vi "Set Output DT.vi"(0 "Scaling configuration in":refnum<class "Scaling configuration.lvclass">, 5 "Scale Data Type":T1, 7 "Scale Index":i32, 9 "Mapping Index":i32, 11 "error in (no error)":errorcluster) -> (4 "Scaling configuration out":refnum<class "Scaling configuration.lvclass">, 15 "error out":errorcluster)   [LabVIEW 2013, in "Scaling configuration.lvclass"]
uses:
  Scaling configuration.lvclass
  controls/scale data types.ctl
  Scaling configuration.lvclass/Scaling configuration.ctl
  <vilib>/NI/Tag Bus/tag/tag descriptor.lvclass/tag descriptor.ctl
  <vilib>/NI/Tag Bus/tag/tag descriptor.lvclass
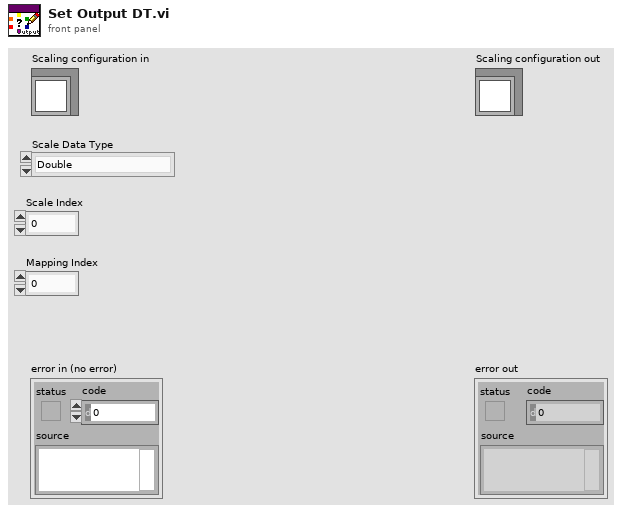
[diagram p1: front panel]
types:
  T1 = typedef "Scaling configuration.lvclass/scale data types.ctl" = enum16{"Double", "Single", "I64", "I32", "I16", "I8", "U64", "U32", "U16", "U8", "Boolean (0,1)"}
  T2 = cluster{"mappings":cluster{"input channel":refnum<class "TBM channel.lvclass">, "output channel":refnum<class "TBM channel.lvclass">, "input data type":T1, "output data type":T1}[], "name":string}[]
  T3 = cluster{"mappings":cluster{"input channel":refnum<class "TBM channel.lvclass">, "output channel":refnum<class "TBM channel.lvclass">, "input data type":T1, "output data type":T1}[], "name":string}
  T4 = cluster{"input channel":refnum<class "TBM channel.lvclass">, "output channel":refnum<class "TBM channel.lvclass">, "input data type":T1, "output data type":T1}[]
  T5 = cluster{"input channel":refnum<class "TBM channel.lvclass">, "output channel":refnum<class "TBM channel.lvclass">, "input data type":T1, "output data type":T1}
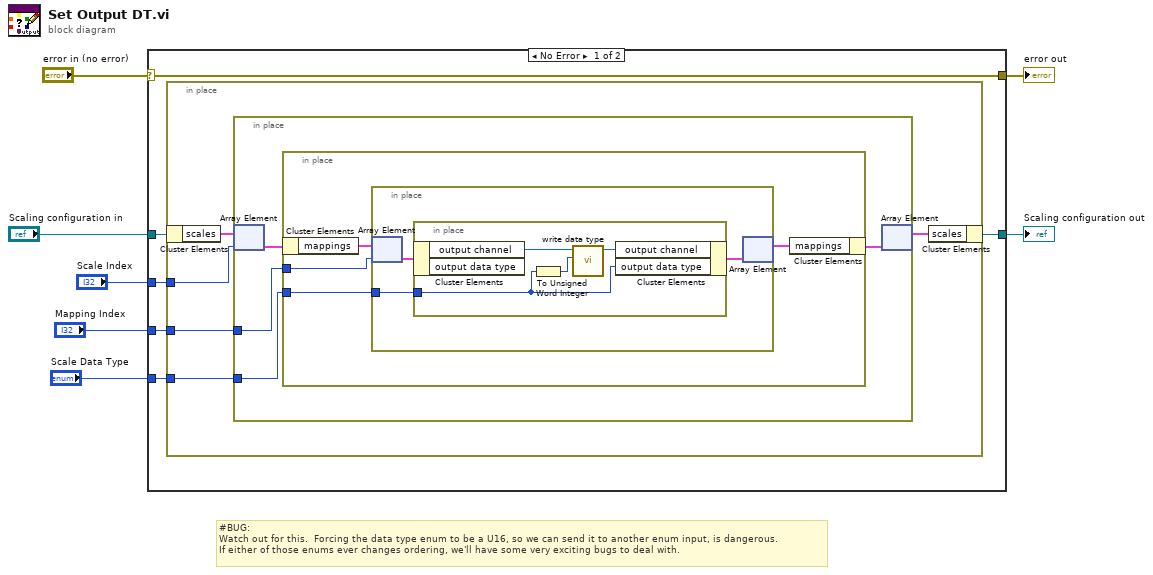
[diagram p0: block diagram]
diagram:
  # "#BUG:\nWatch out for this.  Forcing the data type enum to be a U16, so we can send it to another enum input, is dangerous.\nIf either of those enums ever changes ordering, we'll have some very exciting bugs to deal with."
  n1 = case shown="No Error" "error in (no error)" {
    selector: "error in (no error)" -> [w13 w35]
    tunnel: [w13 w35] -> w6
    tunnel: [w10 w34] -> w4
    tunnel: "Scaling configuration in" -> [w12 w34]
    tunnel: "Scale Index" -> [w11 _]
    tunnel: "Mapping Index" -> [w9 _]
    tunnel: "Scale Data Type" -> [w8 _]
    frame No Error {
      n2 = in-place {
        in-place-border: w11 -> [w17]
        in-place-border: w9 -> [w15]
        in-place-border: w8 -> [w14]
        n3 = in-place-cluster #1(w12) -> ("scales"=w18:T2)
        n4 = in-place {
          in-place-border: w15 -> [w20]
          in-place-border: w14 -> [w19]
          n5 = in-place-array #2(w18, w17) -> (w22:T3)
          n6 = in-place {
            in-place-border: w20 -> [w24]
            in-place-border: w19 -> [w23]
            n7 = in-place-cluster #3(w22) -> ("mappings"=w26:T4)
            n8 = in-place {
              in-place-border: w23 -> [w28]
              n9 = in-place-array #4(w26, w24) -> (w29:T5)
              n10 = in-place {
                in-place-border: w28 -> [w30]
                n11 = in-place-cluster #5(w29) -> ("output channel"=w33:refnum<class "TBM channel.lvclass">)  [unwired: 1 out]
                n12 = To Unsigned Word Integer(number=w30) -> (unsigned 16bit integer=w31:u16)
                n13 = call <vilib>:"write data type.vi"("data type"=w31, "system tag in"=w33) -> ("system tag out"=w32:refnum<class "TBM channel.lvclass">)  [unwired: 8 in, 1 out]
                n14 = in-place-cluster #5("output channel"=w32, "output data type"=w30) -> (w27:T5)
              }
              n15 = in-place-array #4(w27) -> (w25:T4)  [unwired: 1 out]
            }
            n16 = in-place-cluster #3("mappings"=w25) -> (w21:T3)
          }
          n17 = in-place-array #2(w21) -> (w16:T2)  [unwired: 1 out]
        }
        n18 = in-place-cluster #1("scales"=w16) -> (w10:refnum<class "Scaling configuration.lvclass">)
      }
    }
    frame Error {
    }
  }
  "error out" <- w6
  "Scaling configuration out" <- w4
